vi "Initialize UI.vi"(8 "error in (no error)":errorcluster, 11 "Application Data in":T1) -> (0 "error out":errorcluster, 3 "Application Data out":T1)   [LabVIEW 2017, in "DSF Simple Explorer.lvlib"]
uses:
  DSF Configuration.llb/DSF Simple Explorer.lvlib
  Application Data.ctl
  Windows/DSF Core.lvlibp/Classes/Configuration/Configuration Session.lvclass
  View Mode.ctl
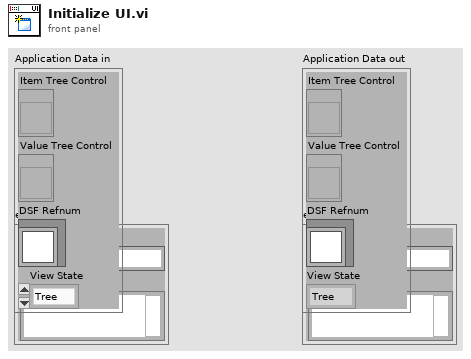
[diagram p1: front panel]
types:
  T1 = typedef "DSF Simple Explorer.lvlib/Application Data.ctl" = cluster{"Item Tree Control":refnum<vi>, "Value Tree Control":refnum<vi>, "DSF Refnum":refnum<class "Configuration Session.lvclass">, "View State":T2}
  T2 = typedef "DSF Simple Explorer.lvlib/View Mode.ctl" = enum16{"Tree", "List"}
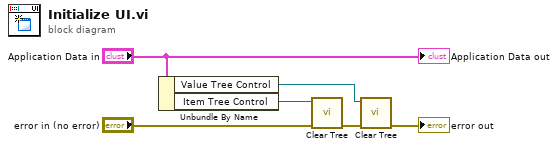
[diagram p0: block diagram]
diagram:
  n1 = Unbundle By Name("Application Data in") -> ("Value Tree Control"=w2:refnum<vi>, "Item Tree Control"=w4:refnum<vi>)
  n2 = call "Clear Tree.vi"("error in (no error)"="error in (no error)", "TreeControl in"=w4) -> ("error out"=w3:errorcluster)  [unwired: 9 in]
  n3 = call "Clear Tree.vi"("error in (no error)"=w3, "TreeControl in"=w2) -> ("error out"=→"error out":errorcluster)  [unwired: 9 in]
  "Application Data out" <- "Application Data in"
